vi "Pass If Error.vi"(7 "Description":string, 8 "error in (no error)":errorcluster, 10 "Assert error":errorcluster, 11 "LUnit Test Case In":refnum<class "LUnit Test Case.lvclass">) -> (0 "error out":errorcluster, 3 "LUnit Test Case Out":refnum<class "LUnit Test Case.lvclass">)   [LabVIEW 2020, in "LUnit Test Case.lvclass"]
doc: "Generates a pass result for the calling test method if the inputs contains an error with status \"True\". A description may be provided to the result."
uses:
  LUnit Test Case.lvclass
  Result/Type.ctl
  LUnit Test Case.lvclass/LUnit Test Case.ctl
  Private/Run In UI.vi
  <vilib>/Utility/error.llb/Clear Errors.vi
  Result/Result.lvlib
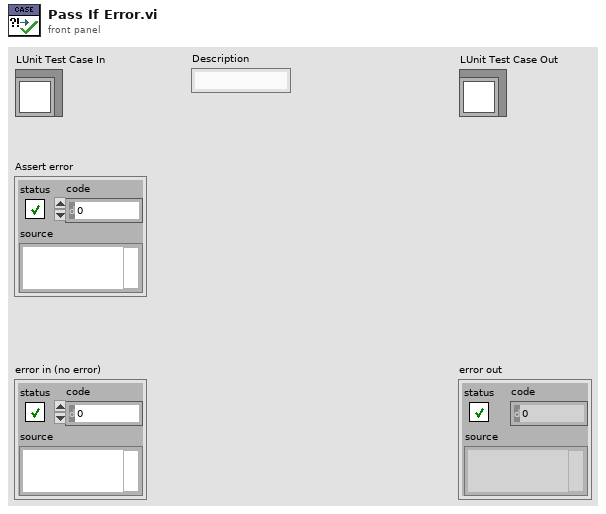
[diagram p1: front panel]
types:
  T1 = typedef "Result.lvlib/Type.ctl" = enum16{"Test Case", "Test Suite", "Test Run", "Pass", "Fail", "Skip", "Pass if", "Fail if", "Pass if Error", "Fail if Error", "Pass if Equal", "Fail if Equal"}
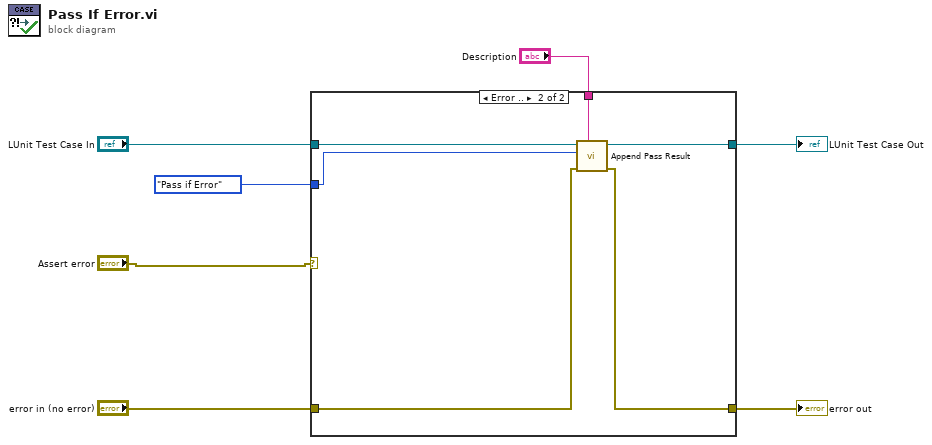
[diagram p0: block diagram]
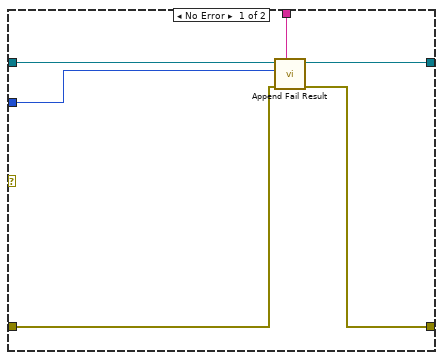
[diagram p2: hidden frame]
diagram:
  n1 = case shown="Error .." "Assert error" {
    tunnel: "LUnit Test Case In" -> [w13 w19]
    tunnel: [w12 w18] -> w6
    tunnel: [w11 w17] -> w5
    tunnel: "Description" -> [w10 w16]
    tunnel: "error in (no error)" -> [w9 w15]
    tunnel: Type."Pass if Error" ("Result Type") -> [w8 w14]
    frame No Error {
      n2 = call "Append Fail Result.vi"("Description"=w10, "error in (no error)"=w9, "Result Type"=w8, "LUnit Test Case In"=w13) -> ("error out"=w11:errorcluster, "LUnit Test Case Out"=w12:refnum<class "LUnit Test Case.lvclass">)  [unwired: 6 in]
    }
    frame Error {
      n3 = call "Append Pass Result.vi"("Description"=w16, "error in (no error)"=w15, "Result Type"=w14, "LUnit Test Case In"=w19) -> ("error out"=w17:errorcluster, "LUnit Test Case Out"=w18:refnum<class "LUnit Test Case.lvclass">)  [unwired: 6 in]
    }
  }
  "error out" <- w5
  "LUnit Test Case Out" <- w6
